vi "mac_db_progress.vi"(8 "error in":errorcluster) -> (0 "error out":errorcluster, 3 "mac_db_lines":i32)   [LabVIEW 2018]
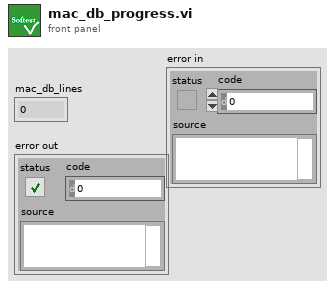
[diagram p1: front panel]
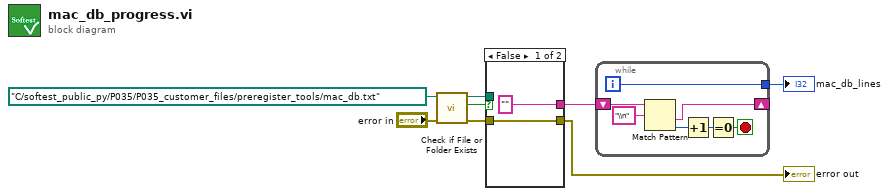
[diagram p0: block diagram]
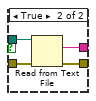
[diagram p2: hidden frame]
diagram:
  n1 = call <vilib>:"Check if File or Folder Exists.vi"("error in (no error)"="error in", "path"=path "C:/softest_public_py/P035/P035_customer_files/preregister_tools/mac_db.txt") -> ("error out"=w7:errorcluster, "file or folder exists?"=w3:bool, "dup path"=w4:path)  [unwired: 7 in]
  n2 = case shown="False" w3 {
    tunnel: w4 -> [_ w14]
    tunnel: ["" w13] -> w5
    tunnel: w7 -> [w9 w12]
    tunnel: [w9 w11] -> w8
    frame False {
    }
    frame True {
      n3 = Read from Text File(file (use dialog)=w14, error in=w12) -> (text=w13:string, error out=w11:errorcluster)  [unwired: 2 in, 2 out]
    }
  }
  "error out" <- w8
  n4 = while {
    shift-right: [w19] -> _
    shift-left: w5 -> [w21]
    tunnel: [w15] -> w6
    i -> [w15]
    stop <- w16 stop-if-true
    n5 = Match Pattern(string=w21, regular expression="\\n") -> (after substring=w19:string, offset past match=w18:i32)  [unwired: 1 in, 2 out]
    n6 = Increment(x=w18) -> (x+1=w17:i32)
    n7 = Equal To 0?(x=w17) -> (x = 0?=w16:bool)
  }
  "mac_db_lines" <- w6
